vi "Application_setValueInViControlByName.vi"(0 "reference":refnum<vi>, 2 "Value":string, 3 "ControlLabel":string="Name", 5 "error in (no error)":errorcluster) -> (14 "reference out":refnum<vi>, 19 "error out":errorcluster)   [LabVIEW 2016]
doc: "Setzt das Objekt mit dem Namen \"Name\" auf den Wert Value\n\n5.6.14 / sige"
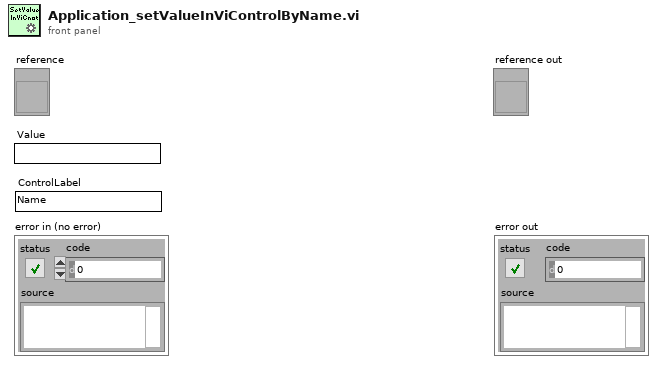
[diagram p1: front panel]
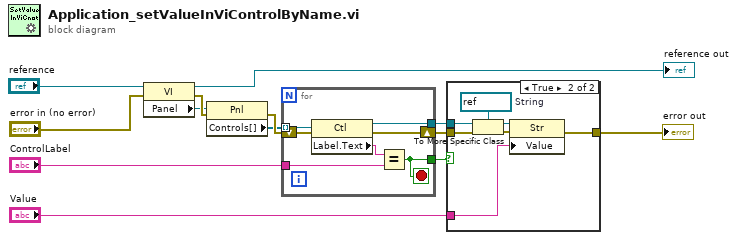
[diagram p0: block diagram]
diagram:
  n1 = property class="VI"(reference="reference", error in="error in (no error)") -> (reference out=→"reference out":refnum<vi>, error out=w8:errorcluster, "Panel"=w5:refnum<vi>)
  n2 = property class="Pnl"(reference=w5, error in=w8) -> (error out=w9:errorcluster, "Controls[]"=w6:refnum<vi>[])  [unwired: 1 out]
  n3 = for {
    tunnel: w6 -> [w20] mode=indexing
    tunnel: [w18] -> w7
    shift-right: [w16] -> w10
    shift-left: w9 -> [w17]
    tunnel: [w15] -> w11
    tunnel: "ControlLabel" -> [w14]
    stop <- w15 stop-if-true
    n4 = property class="Ctl"(reference=w20, error in=w17) -> (reference out=w18:refnum<vi>, error out=w16:errorcluster, "Label.Text"=w19:string)
    n5 = Equal?(x=w19, y=w14) -> (x = y?=w15:bool)
  }
  n6 = case shown="True" w11 {
    tunnel: w7 -> [_ w28]
    tunnel: w10 -> [w21 w24]
    tunnel: [w21 w23] -> w12
    tunnel: "Value" -> [_ w22]
    frame False {
    }
    frame True {
      w26 = refnum<vi> refnum  # String
      n7 = To More Specific Class(target class=w26, reference=w28, error in=w24) -> (specific class reference=w27:refnum<vi>, error out=w25:errorcluster)
      n8 = property class="Str"(reference=w27, error in=w25, "Value"=w22) -> (error out=w23:errorcluster)  [unwired: 1 out]
    }
  }
  "error out" <- w12
